vi "Configure Waveform Modulation Type.vi"(8 "error in (no error)":errorcluster, 9 "Modulation Type (0: Amplitude Modulation)":i32(ring) items=["Amplitude Modulation", "Frequency Modulation", "Frequency-Shift Keying Modulation"], 10 "Waveform Generator Number (1: Waveform Generator 1)":i32(ring)=1 items=["Waveform Generator 1"=1], 11 "VISA resource name":refnum<visa-resource-name>) -> (0 "error out":errorcluster, 3 "VISA resource name out":refnum<visa-resource-name>)   [LabVIEW 2015, in "Agilent 2000 3000 X-Series.lvlib"]
doc: "Selects the modulation type."
uses:
  Agilent 2000 3000 X-Series.lvlib
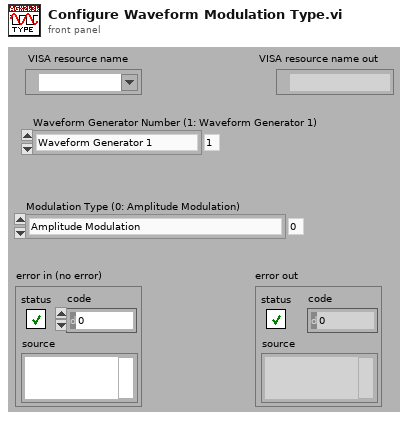
[diagram p1: front panel]
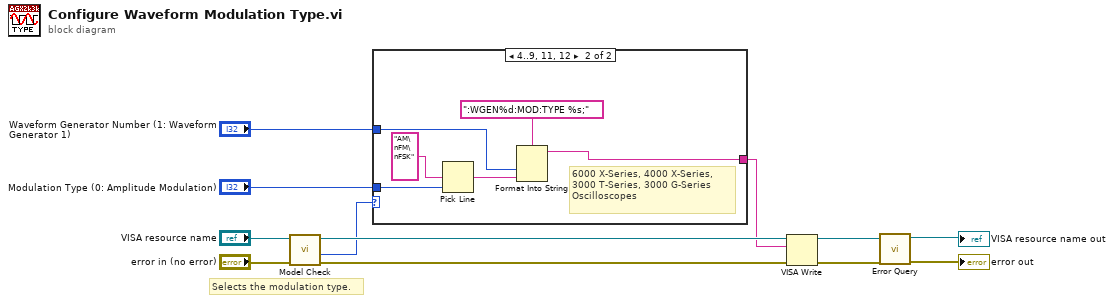
[diagram p0: block diagram]
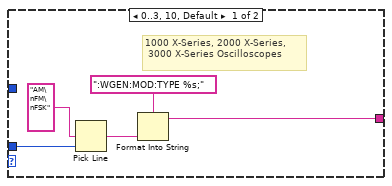
[diagram p2: hidden frame]
diagram:
  # "Selects the modulation type."
  n1 = call "Model Check.vi"("error in (no error)"="error in (no error)", "VISA resource name"="VISA resource name") -> ("error out"=w3:errorcluster, "Model"=w2:i32, "VISA resource name out"=w4:refnum<visa-resource-name>)  [unwired: 7 out]
  n2 = case shown="4..9, 11, 12" w2 {
    tunnel: "Modulation Type (0: Amplitude Modulation)" -> [w16 w20]
    tunnel: "Waveform Generator Number (1: Waveform Generator 1)" -> [_ w19]
    tunnel: [w13 w18] -> w1
    frame 0..3, 10, Default {
      # "1000 X-Series, 2000 X-Series,\n 3000 X-Series Oscilloscopes"
      n3 = Pick Line(multi-line string="AM\nFM\nFSK", line index=w16) -> (output string=w15:string)  [unwired: 1 out]
      n4 = Format Into String(format string=":WGEN:MOD:TYPE %s;", w15) -> (resulting string=w13:string)  [unwired: 2 in, 1 out]
    }
    frame 4..9, 11, 12 {
      # "6000 X-Series, 4000 X-Series, 3000 T-Series, 3000 G-Series  Oscilloscopes"
      n5 = Pick Line(multi-line string="AM\nFM\nFSK", line index=w20) -> (output string=w21:string)  [unwired: 1 out]
      n6 = Format Into String(format string=":WGEN%d:MOD:TYPE %s;", w19, w21) -> (resulting string=w18:string)  [unwired: 2 in, 1 out]
    }
  }
  n7 = VISA Write(VISA resource name=w4, write buffer=w1, error in (no error)=w3) -> (VISA resource name out=w9:refnum<visa-resource-name>, error out=w7:errorcluster)  [unwired: 1 out]
  n8 = call "Error Query.vi"("error in (no error)"=w7, "VISA resource name"=w9) -> ("error out"=→"error out":errorcluster, "VISA resource name out"=→"VISA resource name out":refnum<visa-resource-name>)  [unwired: 6 in, 2 out]
